vi "VISA terminate.vi"(8 "error in (no error)":errorcluster, 11 "Cobolt in":refnum<class "Cobolt.lvclass">) -> (0 "error out":errorcluster, 3 "Cobolt out":refnum<class "Cobolt.lvclass">)   [LabVIEW 2012, in "Cobolt.lvclass"]
uses:
  Cobolt.lvclass
  Cobolt.lvclass/Cobolt.ctl
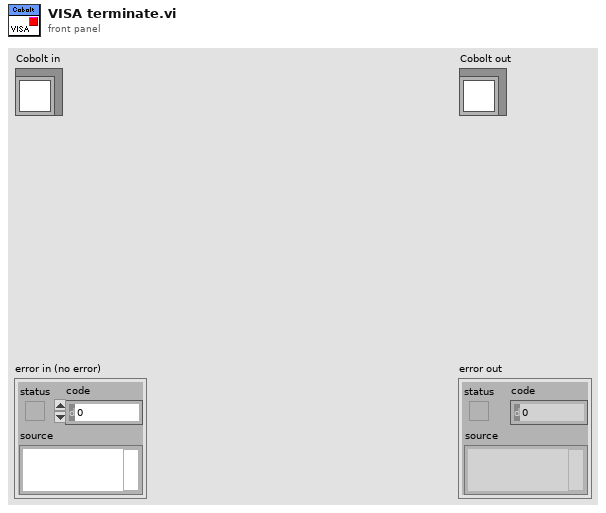
[diagram p1: front panel]
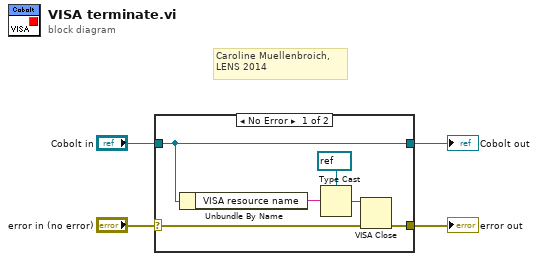
[diagram p0: block diagram]
diagram:
  # "Caroline Muellenbroich, \nLENS 2014"
  n1 = case shown="No Error" "error in (no error)" {
    selector: "error in (no error)" -> [w7 w12]
    tunnel: [w6 w12] -> w3
    tunnel: [w5 w11] -> w1
    tunnel: "Cobolt in" -> [w5 w11]
    frame No Error {
      n2 = Unbundle By Name(w5) -> ("VISA resource name"=w8:string)
      n3 = Type Cast(type=refnum<visa-resource-name> refnum ("VISA resource name"), x=w8) -> (*(type *) &x=w10:refnum<visa-resource-name>)
      n4 = VISA Close(VISA resource name=w10, error in (no error)=w7) -> (error out=w6:errorcluster)
    }
    frame Error {
    }
  }
  "error out" <- w3
  "Cobolt out" <- w1
